vi "CalibrateHeight.vi"(10 "Start Position [mm]":dbl[](array[numeric]), 11 ".NET Refnum In":refnum<k24>) -> (2 "Final Position [mm]":dbl[](array[numeric]))   [LabVIEW 2016]
uses:
  C:/Users/Aerotech/Documents/BNLStaveAssembly-blueprint/Bin/Aerotech.A3200.dll
  BNLStaveAssembly-blueprint/Bin/Aerotech.A3200.dll
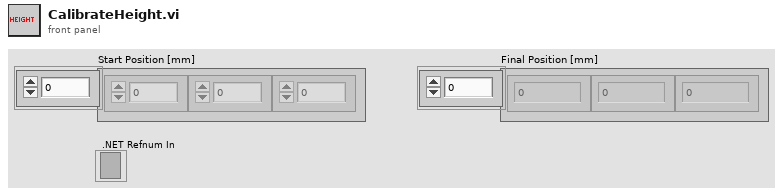
[diagram p1: front panel]
types:
  T1 = cluster{"Final X":dbl, "Final Y":dbl, "Final Z":dbl}
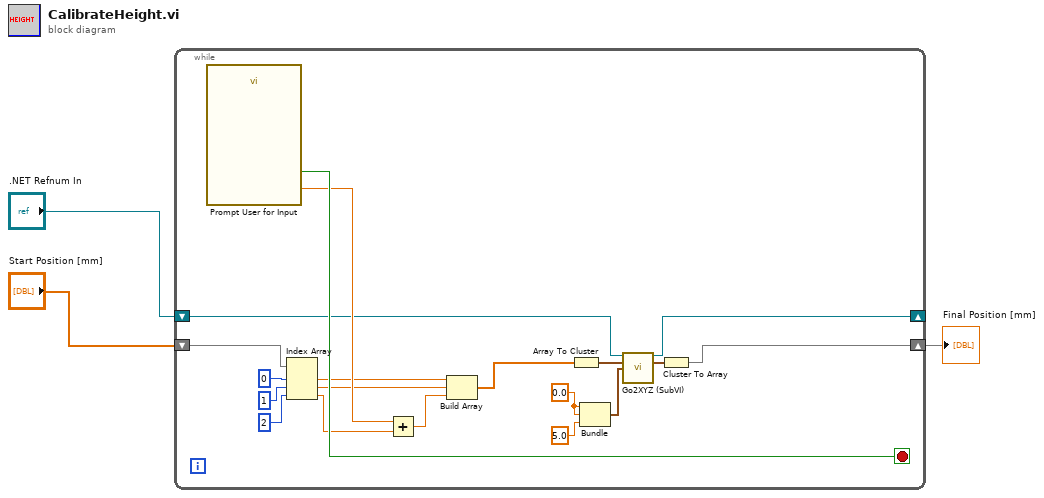
[diagram p0: block diagram]
diagram:
  n1 = while {
    shift-right: [w11] -> w1
    shift-left: "Start Position [mm]" -> [w5]
    shift-right: [w9] -> _
    shift-left: ".NET Refnum In" -> [w10]
    stop <- w22 stop-if-true
    w7 = 0.0
    n2 = call "Prompt User for Input"() -> ("Adjust Height [mm]"=w17:dbl, "Accept"=w22:bool)  [unwired: 16 in, 2 out]
    n3 = Index Array(array=w5, index #1=0 ("index"), index #2=1 ("index"), index #3=2 ("index")) -> (element #1=w14:dbl, element #2=w15:dbl, element #3=w18:dbl)
    n4 = Add(x=w17, y=w18) -> (x+y=w16:dbl)
    n5 = Build Array(w14, w15, w16) -> (w4:dbl[])
    n6 = Array To Cluster(array=w4) -> (cluster=w13:cluster{"[0]":dbl, "[1]":dbl, "[2]":dbl})
    n7 = Bundle(w7, w7, 5.0) -> (w6:cluster{dbl, dbl, dbl})  [unwired: 1 in]
    n8 = call "Go2XYZ (SubVI).vi"(".NET Refnum in"=w10, "Go to Coordinates"=w13, "Axis Speeds"=w6) -> (".NET Refnum out"=w9:refnum<k24>, "Final Position"=w12:T1)  [unwired: 8 in, 3 out]
    n9 = Cluster To Array(cluster=w12) -> (array=w11:dbl[])
  }
  "Final Position [mm]" <- w1
